vi "set_temperature.vi"(1 "PrepLineObject.lvclass":refnum<class "PrepLineObject.lvclass">, 2 "temperature":dbl, 3 "error in (no error)":errorcluster) -> (8 "PrepLineObject out":refnum<class "PrepLineObject.lvclass">, 10 "error out":errorcluster)   [LabVIEW 2017]
doc: "sets the temperature of the instrument that belongs to the PrepLineObject"
uses:
  Classes/PrepLineObject/PrepLineObject.lvclass
  global variables.vi
  Classes/Instrument/instrument.lvclass
  Classes/StatusLog/StatusLog.lvclass
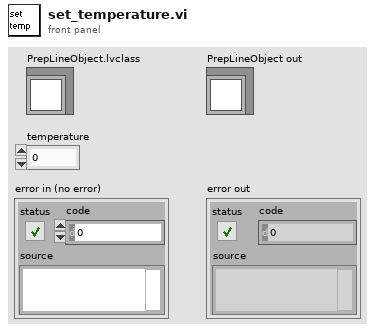
[diagram p1: front panel]
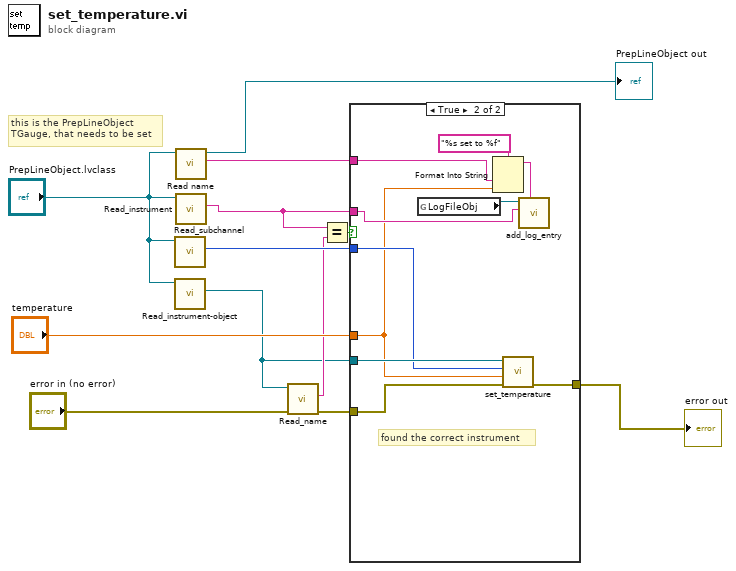
[diagram p0: block diagram]
diagram:
  # "this is the PrepLineObject\nTGauge, that needs to be set"
  n1 = call-dynamic "Read_subchannel.vi"("PrepLineObject in"="PrepLineObject.lvclass") -> ("subchannel"=w10:u16)  [unwired: 8 in, 2 out]
  n2 = call-dynamic "Read_instrument-object.vi"("PrepLineObject in"="PrepLineObject.lvclass") -> ("instrument.lvclass"=w1:refnum<class "instrument.lvclass">)  [unwired: 8 in, 2 out]
  n3 = call-dynamic "Read name.vi"("PrepLineObject in"="PrepLineObject.lvclass") -> ("name"=w7:string, "PrepLineObject out"=→"PrepLineObject out":refnum<class "PrepLineObject.lvclass">)  [unwired: 8 in, 1 out]
  n4 = call-dynamic "Read_instrument.vi"("PrepLinePictureObjects in"="PrepLineObject.lvclass") -> ("instrument name"=w12:string)  [unwired: 7 in, 2 out]
  n5 = call-dynamic "Read_name.vi"("error in (no error)"="error in (no error)", "instrument in"=w1) -> ("error out"=w2:errorcluster, "name"=w4:string)  [unwired: 7 in, 1 out]
  n6 = Equal?(x=w12, y=w4) -> (x = y?=w3:bool)
  n7 = case shown="True" w3 {
    tunnel: w1 -> [_ w21]
    tunnel: w10 -> [_ w20]
    tunnel: "temperature" -> [_ w14]
    tunnel: w2 -> [w13 w23]
    tunnel: [w13 w22] -> w9
    tunnel: w12 -> [_ w16]
    tunnel: w7 -> [_ w15]
    frame False {
      # "wrong instrument"
    }
    frame True {
      # "found the correct instrument"
      n8 = global read "global variables.vi" "LogFileObj"() -> (w19:refnum<class "StatusLog.lvclass">)
      n9 = Format Into String(format string="%s set to %f", w15, w14) -> (resulting string=w18:string)  [unwired: 2 in, 1 out]
      n10 = call-dynamic "set_temperature.vi"("error in (no error)"=w23, "temperature"=w14, "channel"=w20, "instrument in"=w21) -> ("error out"=w22:errorcluster)  [unwired: 6 in, 1 out]
      n11 = call-dynamic "add_log_entry.vi"("new entry"=w18, "log identifiers"=w16, "StatusLog in"=w19) -> ()  [unwired: 5 in, 2 out]
    }
  }
  "error out" <- w9
